vi "Select-U64-hp_state.vi"(10 "hp_state_in":u8[](array[numeric]) format="%.0x", 11 "j":u64) -> (3 "U64(hp_state[j])":u64 format="%.0x")   [LabVIEW 2017]
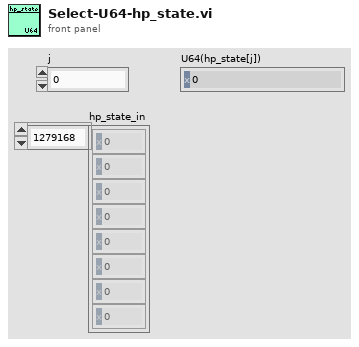
[diagram p1: front panel]
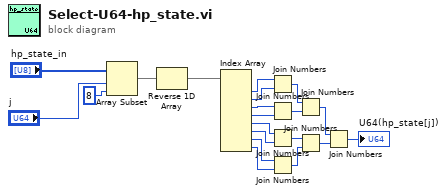
[diagram p0: block diagram]
diagram:
  n1 = Array Subset(array="hp_state_in", index="j", length=8) -> (w5:u8[])
  n2 = Reverse 1D Array(array=w5) -> (reversed array=w1:u8[])
  n3 = Index Array(array=w1) -> (element #1=w13:u8, element #2=w12:u8, element #3=w11:u8, element #4=w10:u8, element #5=w8:u8, element #6=w9:u8, element #7=w7:u8, element #8=w6:u8)  [unwired: 8 in]
  n4 = Join Numbers(hi=w13, lo=w12) -> ((hi.lo)=w17:u16)
  n5 = Join Numbers(hi=w11, lo=w10) -> ((hi.lo)=w16:u16)
  n6 = Join Numbers(hi=w8, lo=w9) -> ((hi.lo)=w15:u16)
  n7 = Join Numbers(hi=w7, lo=w6) -> ((hi.lo)=w14:u16)
  n8 = Join Numbers(hi=w17, lo=w16) -> ((hi.lo)=w18:u32)
  n9 = Join Numbers(hi=w15, lo=w14) -> ((hi.lo)=w19:u32)
  n10 = Join Numbers(hi=w18, lo=w19) -> ((hi.lo)=→"U64(hp_state[j])":u64)
